vi "Find Terminal.vi"(8 "terminal name":string, 11 "Terminals[]":refnum<vi>[](array[refnum])) -> (3 "terminal":refnum<vi>)   [LabVIEW 2020, in "NI_TargetHelper.lvlib"]
uses:
  <vilib>/TargetSupport/NI_TargetHelper/NI_TargetHelper.lvlib
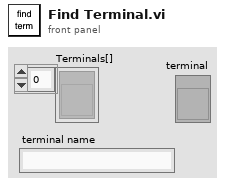
[diagram p1: front panel]
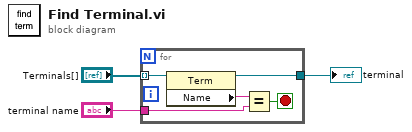
[diagram p0: block diagram]
diagram:
  n1 = for {
    tunnel: "Terminals[]" -> [w8] mode=indexing
    tunnel: [w7] -> w1
    tunnel: "terminal name" -> [w4]
    stop <- w6 stop-if-true
    n2 = property class="Term"(reference=w8) -> (reference out=w7:refnum<vi>, "Name"=w5:string)  [unwired: 1 in, 1 out]
    n3 = Equal?(x=w5, y=w4) -> (x = y?=w6:bool)
  }
  "terminal" <- w1
